vi "ValueWrite1.vi"(2 "Количество знаков после запятой":string, 3 "Ширина строки (в символах)":string, 4 "Файл с заголовком":refnum<file>, 5 "Массив с измерениями":dbl[](array[numeric]), 6 "error in":errorcluster, 7 "Количество датчиков":i32) -> (0 "Файл с заголовком 2":refnum<file>, 1 "error out":errorcluster)   [LabVIEW 2018]
doc: "Производится запись значения величины, поступающего из массива"
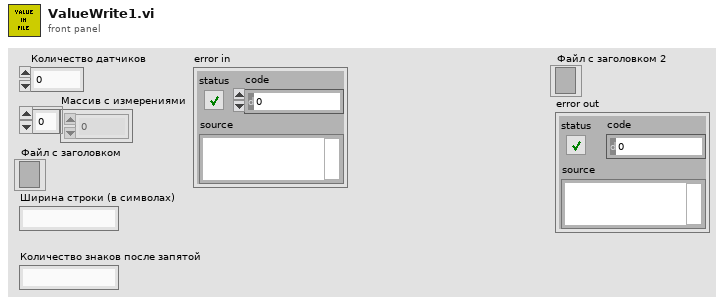
[diagram p1: front panel]
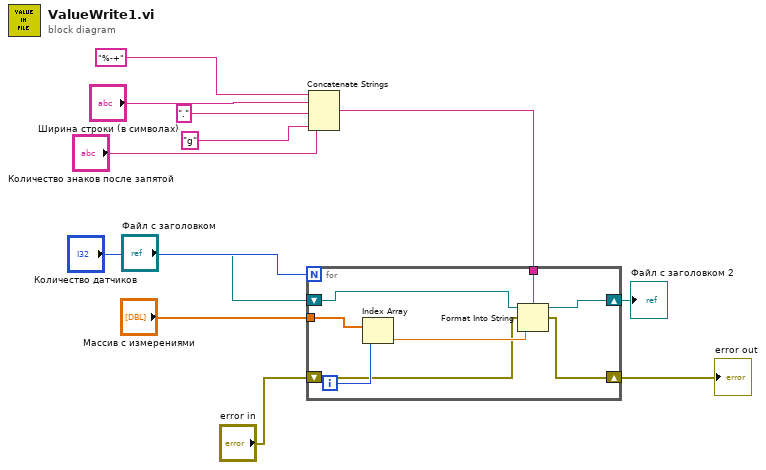
[diagram p0: block diagram]
diagram:
  n1 = Concatenate Strings("%-+" ("string"), "Ширина строки (в символах)", "." ("string"), "Количество знаков после запятой", "g" ("string")) -> (w1:string)
  n2 = for {
    N: "Количество датчиков" -> [_]
    tunnel: "Массив с измерениями" -> [w20]
    shift-right: [w16] -> w9
    shift-left: "Файл с заголовком" -> [w17]
    shift-right: [w14] -> w7
    shift-left: "error in" -> [w15]
    tunnel: w1 -> [w13]
    i -> [w19]
    n3 = Index Array(array=w20, index=w19) -> (element=w18:dbl)
    n4 = Format Into String(format string=w13, initial string=w17, error in=w15, w18) -> (resulting string=w16:refnum<file>, error out=w14:errorcluster)
  }
  "Файл с заголовком 2" <- w9
  "error out" <- w7
